vi "waveform to t-Y cluster (array).vi"(1 "waveform":waveform(dbl)[](array[waveform])) -> (0 "t-Y data":cluster{"t":dbl[], "Y":dbl[]}[](array[cluster]))   [LabVIEW 2010, in "common.lvlib"]
uses:
  common.lvlib
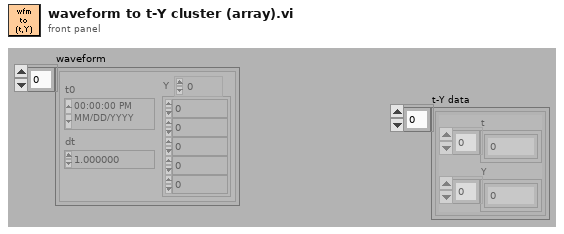
[diagram p1: front panel]
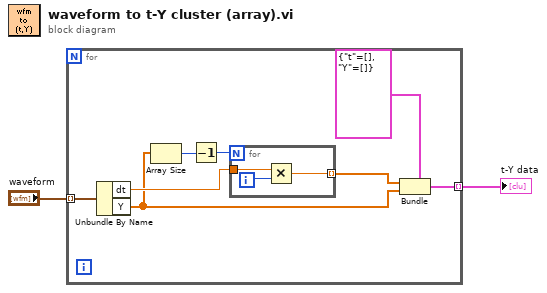
[diagram p0: block diagram]
diagram:
  n1 = for {
    tunnel: "waveform" -> [w9] mode=indexing
    tunnel: [w4] -> w1 mode=indexing
    n2 = Unbundle By Name(w9) -> ("dt"=w10:dbl, "Y"=w5:dbl[])
    n3 = Array Size(array=w5) -> (size(s)=w8:i32)
    n4 = Decrement(x=w8) -> (x-1=w7:i32)
    n5 = for {
      N: w7 -> [_]
      tunnel: w10 -> [w13]
      tunnel: [w11] -> w6 mode=indexing
      i -> [w12]
      n6 = Multiply(x=w13, y=w12) -> (x*y=w11:dbl)
    }
    n7 = Bundle(cluster=cluster{"t":dbl[], "Y":dbl[]} {"t"=[], "Y"=[]} ("t-Y data"), "t"=w6, "Y"=w5) -> (w4:cluster{"t":dbl[], "Y":dbl[]})
  }
  "t-Y data" <- w1
